vi "Collision detect speed test.vi"() -> ()   [LabVIEW 2024]
panel:
  in  "stop":bool
  out "Hz":dbl
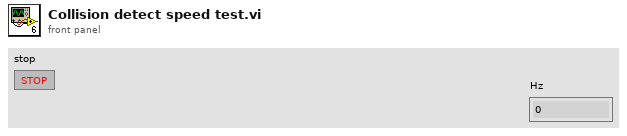
[diagram p1: front panel]
types:
  T1 = cluster{"X":dbl, "Y":dbl, "Object type":dbl, "Move info":dbl, "Vector scalar":dbl, "Vector theta":dbl}
  T2 = cluster{"X":dbl, "Y":dbl, "Object type":dbl, "Radius":dbl, "Width":dbl, "Height":dbl, "Theta":dbl, "HP":dbl, "R":dbl, "G":dbl, "B":dbl}[]
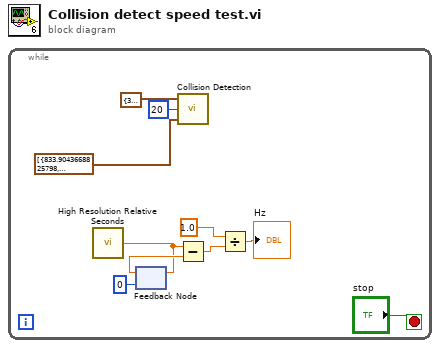
[diagram p0: block diagram]
diagram:
  n1 = while {
    stop <- "stop" stop-if-true
    n2 = call <vilib>:"High Resolution Relative Seconds.vi"() -> ("relative seconds"=w5:dbl)
    n3 = feedback #1(u32 0 ("millisecond timer value")) -> (w6:dbl)
    n4 = feedback-in #1(w5) -> ()
    n5 = call "Collision Detection.vi"("Map Entity Objects Positions"=T2 [{"X"=833.9043668825798, "Y"=359.94566828958796, "Object type"=0.0, "Radius"=30.0, "Width"=0.0, "Height"=0.0, "Theta"=5.711847827345959, "HP"=300.0, "R"=0.0, "G"=0.0, "B"=0.0}, {"X"=2580.0, "Y"=150.0, "Object type"=0.0, "Radius"=30.0, "Width"=0.0, "Height"=0.0, "Theta"=0.0, "HP"=300.0, "R"=0.0, "G"=0.0, "B"=0.0}, {"X"=1470.0, "Y"=390.0, "Object type"=0.0, "Radius"=30.0, "Width"=0.0, "Height"=0.0, "Theta"=0.0, "HP"=300.0, "R"=0.0, "G"=0.0, "B"=0.0}, {"X"=3690.0, "Y"=450.0, "Object type"=0.0, "Radius"=30.0, "Width"=0.0, "Height"=0.0, "Theta"=0.0, "HP"=300.0, "R"=0.0, "G"=0.0, "B"=0.0}, {"X"=2970.0, "Y"=690.0, "Object type"=0.0, "Radius"=30.0, "Width"=0.0, "Height"=0.0, "Theta"=0.0, "HP"=300.0, "R"=0.0, "G"=0.0, "B"=0.0}, {"X"=2130.0, "Y"=750.0, "Object type"=0.0, "Radius"=30.0, "Width"=0.0, "Height"=0.0, "Theta"=0.0, "HP"=300.0, "R"=0.0, "G"=0.0, "B"=0.0}, {"X"=150.0, "Y"=810.0, "Object type"=0.0, "Radius"=30.0, "Width"=0.0, "Height"=0.0, "Theta"=0.0, "HP"=300.0, "R"=0.0, "G"=0.0, "B"=0.0}, {"X"=1290.0, "Y"=1170.0, "Object type"=0.0, "Radius"=30.0, "Width"=0.0, "Height"=0.0, "Theta"=0.0, "HP"=300.0, "R"=0.0, "G"=0.0, "B"=0.0}, {"X"=390.0, "Y"=1290.0, "Object type"=0.0, "Radius"=30.0, "Width"=0.0, "Height"=0.0, "Theta"=0.0, "HP"=300.0, "R"=0.0, "G"=0.0, "B"=0.0}, {"X"=3210.0, "Y"=1290.0, "Object type"=0.0, "Radius"=30.0, "Width"=0.0, "Height"=0.0, "Theta"=0.0, "HP"=300.0, "R"=0.0, "G"=0.0, "B"=0.0}, {"X"=1950.0, "Y"=1710.0, "Object type"=0.0, "Radius"=30.0, "Width"=0.0, "Height"=0.0, "Theta"=0.0, "HP"=300.0, "R"=0.0, "G"=0.0, "B"=0.0}, {"X"=210.0, "Y"=1890.0, "Object type"=0.0, "Radius"=30.0, "Width"=0.0, "Height"=0.0, "Theta"=0.0, "HP"=300.0, "R"=0.0, "G"=0.0, "B"=0.0}, {"X"=2430.0, "Y"=2010.0, "Object type"=0.0, "Radius"=30.0, "Width"=0.0, "Height"=0.0, "Theta"=0.0, "HP"=300.0, "R"=0.0, "G"=0.0, "B"=0.0}, {"X"=3510.0, "Y"=2220.0, "Object type"=0.0, "Radius"=30.0, "Width"=0.0, "Height"=0.0, "Theta"=0.0, "HP"=300.0, "R"=0.0, "G"=0.0, "B"=0.0}, {"X"=1350.0, "Y"=2340.0, "Object type"=0.0, "Radius"=30.0, "Width"=0.0, "Height"=0.0, "Theta"=0.0, "HP"=300.0, "R"=0.0, "G"=0.0, "B"=0.0}, {"X"=330.0, "Y"=2730.0, "Object type"=0.0, "Radius"=30.0, "Width"=0.0, "Height"=0.0, "Theta"=0.0, "HP"=300.0, "R"=0.0, "G"=0.0, "B"=0.0}, {"X"=2790.0, "Y"=2790.0, "Object type"=0.0, "Radius"=30.0, "Width"=0.0, "Height"=0.0, "Theta"=0.0, "HP"=300.0, "R"=0.0, "G"=0.0, "B"=0.0}, {"X"=1950.0, "Y"=3150.0, "Object type"=0.0, "Radius"=30.0, "Width"=0.0, "Height"=0.0, "Theta"=0.0, "HP"=300.0, "R"=0.0, "G"=0.0, "B"=0.0}, {"X"=3330.0, "Y"=3390.0, "Object type"=0.0, "Radius"=30.0, "Width"=0.0, "Height"=0.0, "Theta"=0.0, "HP"=300.0, "R"=0.0, "G"=0.0, "B"=0.0}, {"X"=990.0, "Y"=3450.0, "Object type"=0.0, "Radius"=30.0, "Width"=0.0, "Height"=0.0, "Theta"=0.0, "HP"=300.0, "R"=0.0, "G"=0.0, "B"=0.0}, {"X"=630.0, "Y"=510.0, "Object type"=3.0, "Radius"=47.0, "Width"=0.0, "Height"=0.0, "Theta"=0.0, "HP"=-1000.0, "R"=0.0, "G"=85.0, "B"=0.0}, {"X"=1540.0, "Y"=1054.0, "Object type"=3.0, "Radius"=86.0, "Width"=0.0, "Height"=0.0, "Theta"=0.0, "HP"=-1000.0, "R"=0.0, "G"=85.0, "B"=0.0}, {"X"=1060.0, "Y"=200.0, "Object type"=3.0, "Radius"=72.0, "Width"=0.0, "Height"=0.0, "Theta"=0.0, "HP"=-1000.0, "R"=0.0, "G"=85.0, "B"=0.0}, {"X"=200.0, "Y"=460.0, "Object type"=3.0, "Radius"=62.0, "Width"=0.0, "Height"=0.0, "Theta"=0.0, "HP"=-1000.0, "R"=0.0, "G"=85.0, "B"=0.0}, {"X"=925.0, "Y"=990.0, "Object type"=3.0, "Radius"=68.0, "Width"=0.0, "Height"=0.0, "Theta"=0.0, "HP"=-1000.0, "R"=0.0, "G"=85.0, "B"=0.0}, {"X"=324.0, "Y"=846.0, "Object type"=3.0, "Radius"=73.0, "Width"=0.0, "Height"=0.0, "Theta"=0.0, "HP"=-1000.0, "R"=0.0, "G"=85.0, "B"=0.0}, {"X"=589.0, "Y"=1476.0, "Object type"=3.0, "Radius"=54.0, "Width"=0.0, "Height"=0.0, "Theta"=0.0, "HP"=-1000.0, "R"=0.0, "G"=85.0, "B"=0.0}, {"X"=1650.0, "Y"=1590.0, "Object type"=3.0, "Radius"=60.0, "Width"=0.0, "Height"=0.0, "Theta"=0.0, "HP"=-1000.0, "R"=0.0, "G"=85.0, "B"=0.0}, {"X"=2150.0, "Y"=1590.0, "Object type"=3.0, "Radius"=50.0, "Width"=0.0, "Height"=0.0, "Theta"=0.0, "HP"=-1000.0, "R"=0.0, "G"=85.0, "B"=0.0}, {"X"=990.0, "Y"=690.0, "Object type"=3.0, "Radius"=65.0, "Width"=0.0, "Height"=0.0, "Theta"=0.0, "HP"=-1000.0, "R"=0.0, "G"=85.0, "B"=0.0}, {"X"=1830.0, "Y"=390.0, "Object type"=3.0, "Radius"=73.0, "Width"=0.0, "Height"=0.0, "Theta"=0.0, "HP"=-1000.0, "R"=0.0, "G"=85.0, "B"=0.0}, {"X"=1770.0, "Y"=570.0, "Object type"=3.0, "Radius"=83.0, "Width"=0.0, "Height"=0.0, "Theta"=0.0, "HP"=-1000.0, "R"=0.0, "G"=85.0, "B"=0.0}, {"X"=1950.0, "Y"=510.0, "Object type"=3.0, "Radius"=80.0, "Width"=0.0, "Height"=0.0, "Theta"=0.0, "HP"=-1000.0, "R"=0.0, "G"=85.0, "B"=0.0}, {"X"=201.0, "Y"=140.0, "Object type"=3.0, "Radius"=35.0, "Width"=0.0, "Height"=0.0, "Theta"=0.0, "HP"=-1000.0, "R"=0.0, "G"=255.0, "B"=36.0}, {"X"=340.0, "Y"=160.0, "Object type"=3.0, "Radius"=40.0, "Width"=0.0, "Height"=0.0, "Theta"=0.0, "HP"=-1000.0, "R"=0.0, "G"=255.0, "B"=36.0}, {"X"=2398.0, "Y"=165.0, "Object type"=3.0, "Radius"=37.0, "Width"=0.0, "Height"=0.0, "Theta"=0.0, "HP"=-1000.0, "R"=0.0, "G"=255.0, "B"=36.0}, {"X"=627.0, "Y"=744.0, "Object type"=3.0, "Radius"=21.0, "Width"=0.0, "Height"=0.0, "Theta"=0.0, "HP"=-1000.0, "R"=0.0, "G"=255.0, "B"=36.0}, {"X"=3302.0, "Y"=167.0, "Object type"=3.0, "Radius"=26.0, "Width"=0.0, "Height"=0.0, "Theta"=0.0, "HP"=-1000.0, "R"=0.0, "G"=255.0, "B"=36.0}, {"X"=3587.0, "Y"=199.0, "Object type"=3.0, "Radius"=41.0, "Width"=0.0, "Height"=0.0, "Theta"=0.0, "HP"=-1000.0, "R"=0.0, "G"=255.0, "B"=36.0}, {"X"=3204.0, "Y"=641.0, "Object type"=3.0, "Radius"=33.0, "Width"=0.0, "Height"=0.0, "Theta"=0.0, "HP"=-1000.0, "R"=0.0, "G"=255.0, "B"=36.0}, {"X"=2563.0, "Y"=681.0, "Object type"=3.0, "Radius"=28.0, "Width"=0.0, "Height"=0.0, "Theta"=0.0, "HP"=-1000.0, "R"=0.0, "G"=255.0, "B"=36.0}, {"X"=2913.0, "Y"=867.0, "Object type"=3.0, "Radius"=52.0, "Width"=0.0, "Height"=0.0, "Theta"=0.0, "HP"=-1000.0, "R"=0.0, "G"=255.0, "B"=36.0}, {"X"=3411.0, "Y"=1021.0, "Object type"=3.0, "Radius"=85.0, "Width"=0.0, "Height"=0.0, "Theta"=0.0, "HP"=-1000.0, "R"=0.0, "G"=255.0, "B"=36.0}, {"X"=2453.0, "Y"=941.0, "Object type"=3.0, "Radius"=35.0, "Width"=0.0, "Height"=0.0, "Theta"=0.0, "HP"=-1000.0, "R"=0.0, "G"=255.0, "B"=36.0}, {"X"=2193.0, "Y"=1012.0, "Object type"=3.0, "Radius"=24.0, "Width"=0.0, "Height"=0.0, "Theta"=0.0, "HP"=-1000.0, "R"=179.0, "G"=255.0, "B"=42.0}, {"X"=2134.0, "Y"=1254.0, "Object type"=3.0, "Radius"=34.0, "Width"=0.0, "Height"=0.0, "Theta"=0.0, "HP"=-1000.0, "R"=179.0, "G"=255.0, "B"=42.0}, {"X"=881.0, "Y"=1245.0, "Object type"=3.0, "Radius"=28.0, "Width"=0.0, "Height"=0.0, "Theta"=0.0, "HP"=-1000.0, "R"=179.0, "G"=255.0, "B"=42.0}, {"X"=1000.0, "Y"=1369.0, "Object type"=3.0, "Radius"=32.0, "Width"=0.0, "Height"=0.0, "Theta"=0.0, "HP"=-1000.0, "R"=0.0, "G"=255.0, "B"=36.0}, {"X"=1151.0, "Y"=1489.0, "Object type"=3.0, "Radius"=36.0, "Width"=0.0, "Height"=0.0, "Theta"=0.0, "HP"=-1000.0, "R"=179.0, "G"=255.0, "B"=42.0}, {"X"=399.0, "Y"=1632.0, "Object type"=3.0, "Radius"=28.0, "Width"=0.0, "Height"=0.0, "Theta"=0.0, "HP"=-1000.0, "R"=179.0, "G"=255.0, "B"=42.0}, {"X"=671.0, "Y"=1711.0, "Object type"=3.0, "Radius"=34.0, "Width"=0.0, "Height"=0.0, "Theta"=0.0, "HP"=-1000.0, "R"=179.0, "G"=255.0, "B"=42.0}, {"X"=1025.0, "Y"=1678.0, "Object type"=3.0, "Radius"=36.0, "Width"=0.0, "Height"=0.0, "Theta"=0.0, "HP"=-1000.0, "R"=0.0, "G"=255.0, "B"=36.0}, {"X"=145.0, "Y"=2031.0, "Object type"=3.0, "Radius"=41.0, "Width"=0.0, "Height"=0.0, "Theta"=0.0, "HP"=-1000.0, "R"=0.0, "G"=255.0, "B"=36.0}, {"X"=476.0, "Y"=1931.0, "Object type"=3.0, "Radius"=71.0, "Width"=0.0, "Height"=0.0, "Theta"=0.0, "HP"=-1000.0, "R"=0.0, "G"=255.0, "B"=36.0}, {"X"=756.0, "Y"=1999.0, "Object type"=3.0, "Radius"=29.0, "Width"=0.0, "Height"=0.0, "Theta"=0.0, "HP"=-1000.0, "R"=179.0, "G"=255.0, "B"=42.0}, {"X"=1113.0, "Y"=67.0, "Object type"=3.0, "Radius"=88.0, "Width"=0.0, "Height"=0.0, "Theta"=0.0, "HP"=-1000.0, "R"=0.0, "G"=255.0, "B"=36.0}, {"X"=504.0, "Y"=2241.0, "Object type"=3.0, "Radius"=37.0, "Width"=0.0, "Height"=0.0, "Theta"=0.0, "HP"=-1000.0, "R"=0.0, "G"=255.0, "B"=36.0}, {"X"=936.0, "Y"=2441.0, "Object type"=3.0, "Radius"=25.0, "Width"=0.0, "Height"=0.0, "Theta"=0.0, "HP"=-1000.0, "R"=179.0, "G"=255.0, "B"=42.0}, {"X"=587.0, "Y"=2753.0, "Object type"=3.0, "Radius"=27.0, "Width"=0.0, "Height"=0.0, "Theta"=0.0, "HP"=-1000.0, "R"=179.0, "G"=255.0, "B"=42.0}, {"X"=952.0, "Y"=2801.0, "Object type"=3.0, "Radius"=91.0, "Width"=0.0, "Height"=0.0, "Theta"=0.0, "HP"=-1000.0, "R"=0.0, "G"=255.0, "B"=36.0}, {"X"=134.0, "Y"=3078.0, "Object type"=3.0, "Radius"=67.0, "Width"=0.0, "Height"=0.0, "Theta"=0.0, "HP"=-1000.0, "R"=0.0, "G"=255.0, "B"=36.0}, {"X"=381.0, "Y"=3381.0, "Object type"=3.0, "Radius"=94.0, "Width"=0.0, "Height"=0.0, "Theta"=0.0, "HP"=-1000.0, "R"=179.0, "G"=255.0, "B"=42.0}, {"X"=659.0, "Y"=3549.0, "Object type"=3.0, "Radius"=83.0, "Width"=0.0, "Height"=0.0, "Theta"=0.0, "HP"=-1000.0, "R"=179.0, "G"=255.0, "B"=42.0}, {"X"=921.0, "Y"=3651.0, "Object type"=3.0, "Radius"=33.0, "Width"=0.0, "Height"=0.0, "Theta"=0.0, "HP"=-1000.0, "R"=0.0, "G"=255.0, "B"=36.0}, {"X"=1247.0, "Y"=3539.0, "Object type"=3.0, "Radius"=51.0, "Width"=0.0, "Height"=0.0, "Theta"=0.0, "HP"=-1000.0, "R"=179.0, "G"=255.0, "B"=42.0}, {"X"=1292.0, "Y"=3217.0, "Object type"=3.0, "Radius"=41.0, "Width"=0.0, "Height"=0.0, "Theta"=0.0, "HP"=-1000.0, "R"=0.0, "G"=255.0, "B"=36.0}, {"X"=1435.0, "Y"=2876.0, "Object type"=3.0, "Radius"=79.0, "Width"=0.0, "Height"=0.0, "Theta"=0.0, "HP"=-1000.0, "R"=179.0, "G"=255.0, "B"=42.0}, {"X"=1620.0, "Y"=2173.0, "Object type"=3.0, "Radius"=71.0, "Width"=0.0, "Height"=0.0, "Theta"=0.0, "HP"=-1000.0, "R"=0.0, "G"=255.0, "B"=36.0}, {"X"=1550.0, "Y"=1901.0, "Object type"=3.0, "Radius"=37.0, "Width"=0.0, "Height"=0.0, "Theta"=0.0, "HP"=-1000.0, "R"=0.0, "G"=255.0, "B"=36.0}, {"X"=2786.0, "Y"=1543.0, "Object type"=3.0, "Radius"=26.0, "Width"=0.0, "Height"=0.0, "Theta"=0.0, "HP"=-1000.0, "R"=179.0, "G"=255.0, "B"=42.0}, {"X"=3371.0, "Y"=1701.0, "Object type"=3.0, "Radius"=29.0, "Width"=0.0, "Height"=0.0, "Theta"=0.0, "HP"=-1000.0, "R"=0.0, "G"=255.0, "B"=36.0}, {"X"=3579.0, "Y"=1534.0, "Object type"=3.0, "Radius"=34.0, "Width"=0.0, "Height"=0.0, "Theta"=0.0, "HP"=-1000.0, "R"=179.0, "G"=255.0, "B"=42.0}, {"X"=2482.93, "Y"=321.21, "Object type"=4.0, "Radius"=0.0, "Width"=84.853, "Height"=20.0, "Theta"=2.356, "HP"=-1000.0, "R"=179.0, "G"=255.0, "B"=42.0}, {"X"=2437.07, "Y"=321.21, "Object type"=4.0, "Radius"=0.0, "Width"=84.853, "Height"=20.0, "Theta"=0.785, "HP"=-1000.0, "R"=179.0, "G"=255.0, "B"=42.0}, {"X"=2460.0, "Y"=390.0, "Object type"=4.0, "Radius"=0.0, "Width"=111.72, "Height"=20.0, "Theta"=2.356, "HP"=-1000.0, "R"=179.0, "G"=255.0, "B"=42.0}, {"X"=2482.93, "Y"=458.79, "Object type"=4.0, "Radius"=0.0, "Width"=84.853, "Height"=20.0, "Theta"=0.785, "HP"=-1000.0, "R"=179.0, "G"=255.0, "B"=42.0}, {"X"=2437.07, "Y"=458.79, "Object type"=4.0, "Radius"=0.0, "Width"=84.853, "Height"=20.0, "Theta"=2.356, "HP"=-1000.0, "R"=179.0, "G"=255.0, "B"=42.0}, {"X"=2640.0, "Y"=420.0, "Object type"=4.0, "Radius"=0.0, "Width"=100.0, "Height"=21.0, "Theta"=1.92, "HP"=-1000.0, "R"=179.0, "G"=255.0, "B"=42.0}, {"X"=2700.0, "Y"=420.0, "Object type"=4.0, "Radius"=0.0, "Width"=100.0, "Height"=21.0, "Theta"=1.22, "HP"=-1000.0, "R"=179.0, "G"=255.0, "B"=42.0}, {"X"=2891.0, "Y"=390.0, "Object type"=4.0, "Radius"=0.0, "Width"=120.0, "Height"=18.0, "Theta"=1.57, "HP"=-1000.0, "R"=179.0, "G"=255.0, "B"=42.0}, {"X"=2950.0, "Y"=390.0, "Object type"=4.0, "Radius"=0.0, "Width"=120.0, "Height"=18.0, "Theta"=2.01, "HP"=-1000.0, "R"=179.0, "G"=255.0, "B"=42.0}, {"X"=3060.0, "Y"=390.0, "Object type"=4.0, "Radius"=0.0, "Width"=180.28, "Height"=25.0, "Theta"=1.91, "HP"=-1000.0, "R"=179.0, "G"=255.0, "B"=42.0}, {"X"=3120.0, "Y"=390.0, "Object type"=4.0, "Radius"=0.0, "Width"=180.28, "Height"=25.0, "Theta"=1.23, "HP"=-1000.0, "R"=179.0, "G"=255.0, "B"=42.0}, {"X"=3420.0, "Y"=390.0, "Object type"=4.0, "Radius"=0.0, "Width"=180.28, "Height"=25.0, "Theta"=1.91, "HP"=-1000.0, "R"=179.0, "G"=255.0, "B"=42.0}, {"X"=3480.0, "Y"=390.0, "Object type"=4.0, "Radius"=0.0, "Width"=180.28, "Height"=25.0, "Theta"=1.23, "HP"=-1000.0, "R"=179.0, "G"=255.0, "B"=42.0}, {"X"=435.0, "Y"=260.0, "Object type"=1.0, "Radius"=25.0, "Width"=0.0, "Height"=0.0, "Theta"=0.0, "HP"=-1000.0, "R"=100.0, "G"=60.0, "B"=11.0}, {"X"=1060.0, "Y"=200.0, "Object type"=1.0, "Radius"=23.0, "Width"=0.0, "Height"=0.0, "Theta"=0.0, "HP"=-1000.0, "R"=100.0, "G"=60.0, "B"=11.0}, {"X"=1190.0, "Y"=450.0, "Object type"=1.0, "Radius"=40.0, "Width"=0.0, "Height"=0.0, "Theta"=0.0, "HP"=-1000.0, "R"=100.0, "G"=60.0, "B"=11.0}, {"X"=1300.0, "Y"=670.0, "Object type"=1.0, "Radius"=45.0, "Width"=0.0, "Height"=0.0, "Theta"=0.0, "HP"=-1000.0, "R"=100.0, "G"=60.0, "B"=11.0}, {"X"=200.0, "Y"=460.0, "Object type"=1.0, "Radius"=25.0, "Width"=0.0, "Height"=0.0, "Theta"=0.0, "HP"=-1000.0, "R"=100.0, "G"=60.0, "B"=11.0}, {"X"=630.0, "Y"=470.0, "Object type"=1.0, "Radius"=27.0, "Width"=0.0, "Height"=0.0, "Theta"=0.0, "HP"=-1000.0, "R"=100.0, "G"=60.0, "B"=11.0}, {"X"=575.0, "Y"=543.0, "Object type"=1.0, "Radius"=29.0, "Width"=0.0, "Height"=0.0, "Theta"=0.0, "HP"=-1000.0, "R"=100.0, "G"=60.0, "B"=11.0}, {"X"=660.0, "Y"=554.0, "Object type"=1.0, "Radius"=16.0, "Width"=0.0, "Height"=0.0, "Theta"=0.0, "HP"=-1000.0, "R"=100.0, "G"=60.0, "B"=11.0}, {"X"=329.0, "Y"=846.0, "Object type"=1.0, "Radius"=34.0, "Width"=0.0, "Height"=0.0, "Theta"=0.0, "HP"=-1000.0, "R"=100.0, "G"=60.0, "B"=11.0}, {"X"=621.0, "Y"=883.0, "Object type"=1.0, "Radius"=21.0, "Width"=0.0, "Height"=0.0, "Theta"=0.0, "HP"=-1000.0, "R"=100.0, "G"=60.0, "B"=11.0}, {"X"=925.0, "Y"=990.0, "Object type"=1.0, "Radius"=34.0, "Width"=0.0, "Height"=0.0, "Theta"=0.0, "HP"=-1000.0, "R"=100.0, "G"=60.0, "B"=11.0}, {"X"=1540.0, "Y"=1054.0, "Object type"=1.0, "Radius"=38.0, "Width"=0.0, "Height"=0.0, "Theta"=0.0, "HP"=-1000.0, "R"=100.0, "G"=60.0, "B"=11.0}, {"X"=2940.0, "Y"=145.0, "Object type"=1.0, "Radius"=48.0, "Width"=0.0, "Height"=0.0, "Theta"=0.0, "HP"=-1000.0, "R"=100.0, "G"=60.0, "B"=11.0}, {"X"=167.0, "Y"=1403.0, "Object type"=1.0, "Radius"=29.0, "Width"=0.0, "Height"=0.0, "Theta"=0.0, "HP"=-1000.0, "R"=100.0, "G"=60.0, "B"=11.0}, {"X"=589.0, "Y"=1476.0, "Object type"=1.0, "Radius"=29.0, "Width"=0.0, "Height"=0.0, "Theta"=0.0, "HP"=-1000.0, "R"=100.0, "G"=60.0, "B"=11.0}, {"X"=1650.0, "Y"=1590.0, "Object type"=1.0, "Radius"=27.0, "Width"=0.0, "Height"=0.0, "Theta"=0.0, "HP"=-1000.0, "R"=100.0, "G"=60.0, "B"=11.0}, {"X"=2150.0, "Y"=1950.0, "Object type"=1.0, "Radius"=18.0, "Width"=0.0, "Height"=0.0, "Theta"=0.0, "HP"=-1000.0, "R"=100.0, "G"=60.0, "B"=11.0}, {"X"=1173.0, "Y"=1783.0, "Object type"=1.0, "Radius"=24.0, "Width"=0.0, "Height"=0.0, "Theta"=0.0, "HP"=-1000.0, "R"=100.0, "G"=60.0, "B"=11.0}, {"X"=2261.0, "Y"=1563.0, "Object type"=1.0, "Radius"=31.0, "Width"=0.0, "Height"=0.0, "Theta"=0.0, "HP"=-1000.0, "R"=100.0, "G"=60.0, "B"=11.0}, {"X"=990.0, "Y"=690.0, "Object type"=1.0, "Radius"=32.0, "Width"=0.0, "Height"=0.0, "Theta"=0.0, "HP"=-1000.0, "R"=100.0, "G"=60.0, "B"=11.0}, {"X"=1830.0, "Y"=390.0, "Object type"=1.0, "Radius"=28.0, "Width"=0.0, "Height"=0.0, "Theta"=0.0, "HP"=-1000.0, "R"=100.0, "G"=60.0, "B"=11.0}, {"X"=1770.0, "Y"=570.0, "Object type"=1.0, "Radius"=33.0, "Width"=0.0, "Height"=0.0, "Theta"=0.0, "HP"=-1000.0, "R"=100.0, "G"=60.0, "B"=11.0}, {"X"=1950.0, "Y"=510.0, "Object type"=1.0, "Radius"=36.0, "Width"=0.0, "Height"=0.0, "Theta"=0.0, "HP"=-1000.0, "R"=100.0, "G"=60.0, "B"=11.0}, {"X"=1973.0, "Y"=1121.0, "Object type"=1.0, "Radius"=40.0, "Width"=0.0, "Height"=0.0, "Theta"=0.0, "HP"=-1000.0, "R"=100.0, "G"=60.0, "B"=11.0}, {"X"=2910.0, "Y"=330.0, "Object type"=1.0, "Radius"=28.0, "Width"=0.0, "Height"=0.0, "Theta"=0.0, "HP"=-1000.0, "R"=100.0, "G"=100.0, "B"=100.0}, {"X"=2670.0, "Y"=450.0, "Object type"=1.0, "Radius"=27.0, "Width"=0.0, "Height"=0.0, "Theta"=0.0, "HP"=-1000.0, "R"=100.0, "G"=100.0, "B"=100.0}, {"X"=2173.0, "Y"=378.0, "Object type"=1.0, "Radius"=26.0, "Width"=0.0, "Height"=0.0, "Theta"=0.0, "HP"=-1000.0, "R"=151.0, "G"=151.0, "B"=151.0}, {"X"=3451.0, "Y"=681.0, "Object type"=1.0, "Radius"=32.0, "Width"=0.0, "Height"=0.0, "Theta"=0.0, "HP"=-1000.0, "R"=151.0, "G"=151.0, "B"=151.0}, {"X"=2583.0, "Y"=2927.0, "Object type"=1.0, "Radius"=70.0, "Width"=0.0, "Height"=0.0, "Theta"=0.0, "HP"=-1000.0, "R"=100.0, "G"=100.0, "B"=100.0}, {"X"=2188.0, "Y"=2674.0, "Object type"=1.0, "Radius"=26.0, "Width"=0.0, "Height"=0.0, "Theta"=0.0, "HP"=-1000.0, "R"=151.0, "G"=151.0, "B"=151.0}, {"X"=373.0, "Y"=2539.0, "Object type"=1.0, "Radius"=19.0, "Width"=0.0, "Height"=0.0, "Theta"=0.0, "HP"=-1000.0, "R"=151.0, "G"=151.0, "B"=151.0}, {"X"=256.0, "Y"=2873.0, "Object type"=1.0, "Radius"=14.0, "Width"=0.0, "Height"=0.0, "Theta"=0.0, "HP"=-1000.0, "R"=100.0, "G"=100.0, "B"=100.0}, {"X"=2494.0, "Y"=1248.0, "Object type"=1.0, "Radius"=27.0, "Width"=0.0, "Height"=0.0, "Theta"=0.0, "HP"=-1000.0, "R"=151.0, "G"=151.0, "B"=151.0}, {"X"=814.0, "Y"=2256.0, "Object type"=1.0, "Radius"=45.0, "Width"=0.0, "Height"=0.0, "Theta"=0.0, "HP"=-1000.0, "R"=151.0, "G"=151.0, "B"=151.0}, {"X"=1111.0, "Y"=3345.0, "Object type"=1.0, "Radius"=34.0, "Width"=0.0, "Height"=0.0, "Theta"=0.0, "HP"=-1000.0, "R"=100.0, "G"=100.0, "B"=100.0}, {"X"=3397.0, "Y"=3513.0, "Object type"=2.0, "Radius"=0.0, "Width"=140.0, "Height"=24.0, "Theta"=0.0, "HP"=-1000.0, "R"=100.0, "G"=100.0, "B"=100.0}, {"X"=3510.0, "Y"=3456.0, "Object type"=2.0, "Radius"=0.0, "Width"=120.0, "Height"=37.0, "Theta"=0.96, "HP"=-1000.0, "R"=100.0, "G"=100.0, "B"=100.0}, {"X"=3176.0, "Y"=3238.0, "Object type"=2.0, "Radius"=0.0, "Width"=137.0, "Height"=29.0, "Theta"=0.0, "HP"=-1000.0, "R"=151.0, "G"=151.0, "B"=151.0}, {"X"=3382.0, "Y"=3098.0, "Object type"=2.0, "Radius"=0.0, "Width"=163.0, "Height"=33.0, "Theta"=2.18, "HP"=-1000.0, "R"=100.0, "G"=100.0, "B"=100.0}, {"X"=3340.0, "Y"=2120.0, "Object type"=2.0, "Radius"=0.0, "Width"=140.0, "Height"=40.0, "Theta"=1.57, "HP"=-1000.0, "R"=100.0, "G"=100.0, "B"=100.0}, {"X"=3340.0, "Y"=2240.0, "Object type"=2.0, "Radius"=0.0, "Width"=100.0, "Height"=40.0, "Theta"=1.57, "HP"=-1000.0, "R"=100.0, "G"=100.0, "B"=100.0}, {"X"=2140.0, "Y"=1980.0, "Object type"=2.0, "Radius"=0.0, "Width"=160.0, "Height"=20.0, "Theta"=0.0, "HP"=-1000.0, "R"=100.0, "G"=100.0, "B"=100.0}, {"X"=2080.0, "Y"=1960.0, "Object type"=2.0, "Radius"=0.0, "Width"=160.0, "Height"=20.0, "Theta"=1.57, "HP"=-1000.0, "R"=100.0, "G"=100.0, "B"=100.0}, {"X"=2160.0, "Y"=2020.0, "Object type"=2.0, "Radius"=0.0, "Width"=160.0, "Height"=20.0, "Theta"=0.0, "HP"=-1000.0, "R"=100.0, "G"=100.0, "B"=100.0}, {"X"=2220.0, "Y"=1940.0, "Object type"=2.0, "Radius"=0.0, "Width"=160.0, "Height"=20.0, "Theta"=1.57, "HP"=-1000.0, "R"=100.0, "G"=100.0, "B"=100.0}, {"X"=1592.66, "Y"=1549.85, "Object type"=2.0, "Radius"=0.0, "Width"=160.0, "Height"=20.0, "Theta"=0.96, "HP"=-1000.0, "R"=100.0, "G"=100.0, "B"=100.0}, {"X"=1609.85, "Y"=1647.34, "Object type"=2.0, "Radius"=0.0, "Width"=160.0, "Height"=20.0, "Theta"=2.53, "HP"=-1000.0, "R"=100.0, "G"=100.0, "B"=100.0}, {"X"=1707.34, "Y"=1630.15, "Object type"=2.0, "Radius"=0.0, "Width"=160.0, "Height"=20.0, "Theta"=0.96, "HP"=-1000.0, "R"=100.0, "G"=100.0, "B"=100.0}, {"X"=1690.15, "Y"=1532.66, "Object type"=2.0, "Radius"=0.0, "Width"=160.0, "Height"=20.0, "Theta"=2.53, "HP"=-1000.0, "R"=100.0, "G"=100.0, "B"=100.0}, {"X"=2910.0, "Y"=3150.0, "Object type"=2.0, "Radius"=0.0, "Width"=180.0, "Height"=35.0, "Theta"=1.57, "HP"=-1000.0, "R"=151.0, "G"=151.0, "B"=151.0}, {"X"=2910.0, "Y"=3330.0, "Object type"=2.0, "Radius"=0.0, "Width"=180.0, "Height"=35.0, "Theta"=1.57, "HP"=-1000.0, "R"=151.0, "G"=151.0, "B"=151.0}, {"X"=2600.0, "Y"=3500.0, "Object type"=2.0, "Radius"=0.0, "Width"=170.0, "Height"=25.0, "Theta"=1.8, "HP"=-1000.0, "R"=100.0, "G"=100.0, "B"=100.0}, {"X"=2300.0, "Y"=3535.0, "Object type"=2.0, "Radius"=0.0, "Width"=190.0, "Height"=30.0, "Theta"=0.4, "HP"=-1000.0, "R"=151.0, "G"=151.0, "B"=151.0}, {"X"=2000.0, "Y"=3640.0, "Object type"=2.0, "Radius"=0.0, "Width"=185.0, "Height"=27.0, "Theta"=1.34, "HP"=-1000.0, "R"=100.0, "G"=100.0, "B"=100.0}, {"X"=1730.0, "Y"=3170.0, "Object type"=2.0, "Radius"=0.0, "Width"=195.0, "Height"=33.0, "Theta"=1.77, "HP"=-1000.0, "R"=100.0, "G"=100.0, "B"=100.0}, {"X"=3140.0, "Y"=2785.0, "Object type"=2.0, "Radius"=0.0, "Width"=158.0, "Height"=18.0, "Theta"=1.64, "HP"=-1000.0, "R"=151.0, "G"=151.0, "B"=151.0}, {"X"=2650.0, "Y"=2485.0, "Object type"=2.0, "Radius"=0.0, "Width"=200.0, "Height"=40.0, "Theta"=6.0, "HP"=-1000.0, "R"=100.0, "G"=100.0, "B"=100.0}, {"X"=3014.0, "Y"=2178.0, "Object type"=2.0, "Radius"=0.0, "Width"=175.0, "Height"=22.0, "Theta"=1.14, "HP"=-1000.0, "R"=100.0, "G"=100.0, "B"=100.0}, {"X"=1966.0, "Y"=2498.0, "Object type"=2.0, "Radius"=0.0, "Width"=190.0, "Height"=25.0, "Theta"=1.6, "HP"=-1000.0, "R"=151.0, "G"=151.0, "B"=151.0}, {"X"=867.0, "Y"=3098.0, "Object type"=2.0, "Radius"=0.0, "Width"=187.0, "Height"=24.0, "Theta"=5.91, "HP"=-1000.0, "R"=100.0, "G"=100.0, "B"=100.0}, {"X"=3054.0, "Y"=1154.0, "Object type"=2.0, "Radius"=0.0, "Width"=160.0, "Height"=38.0, "Theta"=5.8, "HP"=-1000.0, "R"=100.0, "G"=100.0, "B"=100.0}, {"X"=3324.0, "Y"=1503.0, "Object type"=2.0, "Radius"=0.0, "Width"=150.0, "Height"=20.0, "Theta"=0.61, "HP"=-1000.0, "R"=151.0, "G"=151.0, "B"=151.0}, {"X"=2301.0, "Y"=3504.0, "Object type"=2.0, "Radius"=0.0, "Width"=145.0, "Height"=24.0, "Theta"=0.85, "HP"=-1000.0, "R"=151.0, "G"=151.0, "B"=151.0}, {"X"=100.0, "Y"=10.0, "Object type"=2.0, "Radius"=0.0, "Width"=200.0, "Height"=20.0, "Theta"=0.0, "HP"=-1000.0, "R"=100.0, "G"=100.0, "B"=100.0}, {"X"=300.0, "Y"=10.0, "Object type"=2.0, "Radius"=0.0, "Width"=200.0, "Height"=20.0, "Theta"=0.0, "HP"=-1000.0, "R"=100.0, "G"=100.0, "B"=100.0}, {"X"=500.0, "Y"=10.0, "Object type"=2.0, "Radius"=0.0, "Width"=200.0, "Height"=20.0, "Theta"=0.0, "HP"=-1000.0, "R"=100.0, "G"=100.0, "B"=100.0}, {"X"=700.0, "Y"=10.0, "Object type"=2.0, "Radius"=0.0, "Width"=200.0, "Height"=20.0, "Theta"=0.0, "HP"=-1000.0, "R"=100.0, "G"=100.0, "B"=100.0}, {"X"=900.0, "Y"=10.0, "Object type"=2.0, "Radius"=0.0, "Width"=200.0, "Height"=20.0, "Theta"=0.0, "HP"=-1000.0, "R"=100.0, "G"=100.0, "B"=100.0}, {"X"=1100.0, "Y"=10.0, "Object type"=2.0, "Radius"=0.0, "Width"=200.0, "Height"=20.0, "Theta"=0.0, "HP"=-1000.0, "R"=100.0, "G"=100.0, "B"=100.0}, {"X"=1300.0, "Y"=10.0, "Object type"=2.0, "Radius"=0.0, "Width"=200.0, "Height"=20.0, "Theta"=0.0, "HP"=-1000.0, "R"=100.0, "G"=100.0, "B"=100.0}, {"X"=1500.0, "Y"=10.0, "Object type"=2.0, "Radius"=0.0, "Width"=200.0, "Height"=20.0, "Theta"=0.0, "HP"=-1000.0, "R"=100.0, "G"=100.0, "B"=100.0}, {"X"=1700.0, "Y"=10.0, "Object type"=2.0, "Radius"=0.0, "Width"=200.0, "Height"=20.0, "Theta"=0.0, "HP"=-1000.0, "R"=100.0, "G"=100.0, "B"=100.0}, {"X"=1900.0, "Y"=10.0, "Object type"=2.0, "Radius"=0.0, "Width"=200.0, "Height"=20.0, "Theta"=0.0, "HP"=-1000.0, "R"=100.0, "G"=100.0, "B"=100.0}, {"X"=2100.0, "Y"=10.0, "Object type"=2.0, "Radius"=0.0, "Width"=200.0, "Height"=20.0, "Theta"=0.0, "HP"=-1000.0, "R"=100.0, "G"=100.0, "B"=100.0}, {"X"=2300.0, "Y"=10.0, "Object type"=2.0, "Radius"=0.0, "Width"=200.0, "Height"=20.0, "Theta"=0.0, "HP"=-1000.0, "R"=100.0, "G"=100.0, "B"=100.0}, {"X"=2500.0, "Y"=10.0, "Object type"=2.0, "Radius"=0.0, "Width"=200.0, "Height"=20.0, "Theta"=0.0, "HP"=-1000.0, "R"=100.0, "G"=100.0, "B"=100.0}, {"X"=2700.0, "Y"=10.0, "Object type"=2.0, "Radius"=0.0, "Width"=200.0, "Height"=20.0, "Theta"=0.0, "HP"=-1000.0, "R"=100.0, "G"=100.0, "B"=100.0}, {"X"=2900.0, "Y"=10.0, "Object type"=2.0, "Radius"=0.0, "Width"=200.0, "Height"=20.0, "Theta"=0.0, "HP"=-1000.0, "R"=100.0, "G"=100.0, "B"=100.0}, {"X"=3100.0, "Y"=10.0, "Object type"=2.0, "Radius"=0.0, "Width"=200.0, "Height"=20.0, "Theta"=0.0, "HP"=-1000.0, "R"=100.0, "G"=100.0, "B"=100.0}, {"X"=3300.0, "Y"=10.0, "Object type"=2.0, "Radius"=0.0, "Width"=200.0, "Height"=20.0, "Theta"=0.0, "HP"=-1000.0, "R"=100.0, "G"=100.0, "B"=100.0}, {"X"=3500.0, "Y"=10.0, "Object type"=2.0, "Radius"=0.0, "Width"=200.0, "Height"=20.0, "Theta"=0.0, "HP"=-1000.0, "R"=100.0, "G"=100.0, "B"=100.0}, {"X"=3700.0, "Y"=10.0, "Object type"=2.0, "Radius"=0.0, "Width"=200.0, "Height"=20.0, "Theta"=0.0, "HP"=-1000.0, "R"=100.0, "G"=100.0, "B"=100.0}, {"X"=3900.0, "Y"=10.0, "Object type"=2.0, "Radius"=0.0, "Width"=200.0, "Height"=20.0, "Theta"=0.0, "HP"=-1000.0, "R"=100.0, "G"=100.0, "B"=100.0}, {"X"=100.0, "Y"=3830.0, "Object type"=2.0, "Radius"=0.0, "Width"=200.0, "Height"=20.0, "Theta"=0.0, "HP"=-1000.0, "R"=100.0, "G"=100.0, "B"=100.0}, {"X"=300.0, "Y"=3830.0, "Object type"=2.0, "Radius"=0.0, "Width"=200.0, "Height"=20.0, "Theta"=0.0, "HP"=-1000.0, "R"=100.0, "G"=100.0, "B"=100.0}, {"X"=500.0, "Y"=3830.0, "Object type"=2.0, "Radius"=0.0, "Width"=200.0, "Height"=20.0, "Theta"=0.0, "HP"=-1000.0, "R"=100.0, "G"=100.0, "B"=100.0}, {"X"=700.0, "Y"=3830.0, "Object type"=2.0, "Radius"=0.0, "Width"=200.0, "Height"=20.0, "Theta"=0.0, "HP"=-1000.0, "R"=100.0, "G"=100.0, "B"=100.0}, {"X"=900.0, "Y"=3830.0, "Object type"=2.0, "Radius"=0.0, "Width"=200.0, "Height"=20.0, "Theta"=0.0, "HP"=-1000.0, "R"=100.0, "G"=100.0, "B"=100.0}, {"X"=1100.0, "Y"=3830.0, "Object type"=2.0, "Radius"=0.0, "Width"=200.0, "Height"=20.0, "Theta"=0.0, "HP"=-1000.0, "R"=100.0, "G"=100.0, "B"=100.0}, {"X"=1300.0, "Y"=3830.0, "Object type"=2.0, "Radius"=0.0, "Width"=200.0, "Height"=20.0, "Theta"=0.0, "HP"=-1000.0, "R"=100.0, "G"=100.0, "B"=100.0}, {"X"=1500.0, "Y"=3830.0, "Object type"=2.0, "Radius"=0.0, "Width"=200.0, "Height"=20.0, "Theta"=0.0, "HP"=-1000.0, "R"=100.0, "G"=100.0, "B"=100.0}, {"X"=1700.0, "Y"=3830.0, "Object type"=2.0, "Radius"=0.0, "Width"=200.0, "Height"=20.0, "Theta"=0.0, "HP"=-1000.0, "R"=100.0, "G"=100.0, "B"=100.0}, {"X"=1900.0, "Y"=3830.0, "Object type"=2.0, "Radius"=0.0, "Width"=200.0, "Height"=20.0, "Theta"=0.0, "HP"=-1000.0, "R"=100.0, "G"=100.0, "B"=100.0}, {"X"=2100.0, "Y"=3830.0, "Object type"=2.0, "Radius"=0.0, "Width"=200.0, "Height"=20.0, "Theta"=0.0, "HP"=-1000.0, "R"=100.0, "G"=100.0, "B"=100.0}, {"X"=2300.0, "Y"=3830.0, "Object type"=2.0, "Radius"=0.0, "Width"=200.0, "Height"=20.0, "Theta"=0.0, "HP"=-1000.0, "R"=100.0, "G"=100.0, "B"=100.0}, {"X"=2500.0, "Y"=3830.0, "Object type"=2.0, "Radius"=0.0, "Width"=200.0, "Height"=20.0, "Theta"=0.0, "HP"=-1000.0, "R"=100.0, "G"=100.0, "B"=100.0}, {"X"=2700.0, "Y"=3830.0, "Object type"=2.0, "Radius"=0.0, "Width"=200.0, "Height"=20.0, "Theta"=0.0, "HP"=-1000.0, "R"=100.0, "G"=100.0, "B"=100.0}, {"X"=2900.0, "Y"=3830.0, "Object type"=2.0, "Radius"=0.0, "Width"=200.0, "Height"=20.0, "Theta"=0.0, "HP"=-1000.0, "R"=100.0, "G"=100.0, "B"=100.0}, {"X"=3100.0, "Y"=3830.0, "Object type"=2.0, "Radius"=0.0, "Width"=200.0, "Height"=20.0, "Theta"=0.0, "HP"=-1000.0, "R"=100.0, "G"=100.0, "B"=100.0}, {"X"=3300.0, "Y"=3830.0, "Object type"=2.0, "Radius"=0.0, "Width"=200.0, "Height"=20.0, "Theta"=0.0, "HP"=-1000.0, "R"=100.0, "G"=100.0, "B"=100.0}, {"X"=3500.0, "Y"=3830.0, "Object type"=2.0, "Radius"=0.0, "Width"=200.0, "Height"=20.0, "Theta"=0.0, "HP"=-1000.0, "R"=100.0, "G"=100.0, "B"=100.0}, {"X"=3700.0, "Y"=3830.0, "Object type"=2.0, "Radius"=0.0, "Width"=200.0, "Height"=20.0, "Theta"=0.0, "HP"=-1000.0, "R"=100.0, "G"=100.0, "B"=100.0}, {"X"=3900.0, "Y"=3830.0, "Object type"=2.0, "Radius"=0.0, "Width"=200.0, "Height"=20.0, "Theta"=0.0, "HP"=-1000.0, "R"=100.0, "G"=100.0, "B"=100.0}, {"X"=10.0, "Y"=120.0, "Object type"=2.0, "Radius"=0.0, "Width"=200.0, "Height"=20.0, "Theta"=1.57, "HP"=-1000.0, "R"=100.0, "G"=100.0, "B"=100.0}, {"X"=10.0, "Y"=320.0, "Object type"=2.0, "Radius"=0.0, "Width"=200.0, "Height"=20.0, "Theta"=1.57, "HP"=-1000.0, "R"=100.0, "G"=100.0, "B"=100.0}, {"X"=10.0, "Y"=520.0, "Object type"=2.0, "Radius"=0.0, "Width"=200.0, "Height"=20.0, "Theta"=1.57, "HP"=-1000.0, "R"=100.0, "G"=100.0, "B"=100.0}, {"X"=10.0, "Y"=720.0, "Object type"=2.0, "Radius"=0.0, "Width"=200.0, "Height"=20.0, "Theta"=1.57, "HP"=-1000.0, "R"=100.0, "G"=100.0, "B"=100.0}, {"X"=10.0, "Y"=920.0, "Object type"=2.0, "Radius"=0.0, "Width"=200.0, "Height"=20.0, "Theta"=1.57, "HP"=-1000.0, "R"=100.0, "G"=100.0, "B"=100.0}, {"X"=10.0, "Y"=1120.0, "Object type"=2.0, "Radius"=0.0, "Width"=200.0, "Height"=20.0, "Theta"=1.57, "HP"=-1000.0, "R"=100.0, "G"=100.0, "B"=100.0}, {"X"=10.0, "Y"=1320.0, "Object type"=2.0, "Radius"=0.0, "Width"=200.0, "Height"=20.0, "Theta"=1.57, "HP"=-1000.0, "R"=100.0, "G"=100.0, "B"=100.0}, {"X"=10.0, "Y"=1520.0, "Object type"=2.0, "Radius"=0.0, "Width"=200.0, "Height"=20.0, "Theta"=1.57, "HP"=-1000.0, "R"=100.0, "G"=100.0, "B"=100.0}, {"X"=10.0, "Y"=1720.0, "Object type"=2.0, "Radius"=0.0, "Width"=200.0, "Height"=20.0, "Theta"=1.57, "HP"=-1000.0, "R"=100.0, "G"=100.0, "B"=100.0}, {"X"=10.0, "Y"=1920.0, "Object type"=2.0, "Radius"=0.0, "Width"=200.0, "Height"=20.0, "Theta"=1.57, "HP"=-1000.0, "R"=100.0, "G"=100.0, "B"=100.0}, {"X"=10.0, "Y"=2120.0, "Object type"=2.0, "Radius"=0.0, "Width"=200.0, "Height"=20.0, "Theta"=1.57, "HP"=-1000.0, "R"=100.0, "G"=100.0, "B"=100.0}, {"X"=10.0, "Y"=2320.0, "Object type"=2.0, "Radius"=0.0, "Width"=200.0, "Height"=20.0, "Theta"=1.57, "HP"=-1000.0, "R"=100.0, "G"=100.0, "B"=100.0}, {"X"=10.0, "Y"=2520.0, "Object type"=2.0, "Radius"=0.0, "Width"=200.0, "Height"=20.0, "Theta"=1.57, "HP"=-1000.0, "R"=100.0, "G"=100.0, "B"=100.0}, {"X"=10.0, "Y"=2720.0, "Object type"=2.0, "Radius"=0.0, "Width"=200.0, "Height"=20.0, "Theta"=1.57, "HP"=-1000.0, "R"=100.0, "G"=100.0, "B"=100.0}, {"X"=10.0, "Y"=2920.0, "Object type"=2.0, "Radius"=0.0, "Width"=200.0, "Height"=20.0, "Theta"=1.57, "HP"=-1000.0, "R"=100.0, "G"=100.0, "B"=100.0}, {"X"=10.0, "Y"=3120.0, "Object type"=2.0, "Radius"=0.0, "Width"=200.0, "Height"=20.0, "Theta"=1.57, "HP"=-1000.0, "R"=100.0, "G"=100.0, "B"=100.0}, {"X"=10.0, "Y"=3320.0, "Object type"=2.0, "Radius"=0.0, "Width"=200.0, "Height"=20.0, "Theta"=1.57, "HP"=-1000.0, "R"=100.0, "G"=100.0, "B"=100.0}, {"X"=10.0, "Y"=3520.0, "Object type"=2.0, "Radius"=0.0, "Width"=200.0, "Height"=20.0, "Theta"=1.57, "HP"=-1000.0, "R"=100.0, "G"=100.0, "B"=100.0}, {"X"=10.0, "Y"=3720.0, "Object type"=2.0, "Radius"=0.0, "Width"=200.0, "Height"=20.0, "Theta"=1.57, "HP"=-1000.0, "R"=100.0, "G"=100.0, "B"=100.0}, {"X"=3830.0, "Y"=120.0, "Object type"=2.0, "Radius"=0.0, "Width"=200.0, "Height"=20.0, "Theta"=1.57, "HP"=-1000.0, "R"=100.0, "G"=100.0, "B"=100.0}, {"X"=3830.0, "Y"=320.0, "Object type"=2.0, "Radius"=0.0, "Width"=200.0, "Height"=20.0, "Theta"=1.57, "HP"=-1000.0, "R"=100.0, "G"=100.0, "B"=100.0}, {"X"=3830.0, "Y"=520.0, "Object type"=2.0, "Radius"=0.0, "Width"=200.0, "Height"=20.0, "Theta"=1.57, "HP"=-1000.0, "R"=100.0, "G"=100.0, "B"=100.0}, {"X"=3830.0, "Y"=720.0, "Object type"=2.0, "Radius"=0.0, "Width"=200.0, "Height"=20.0, "Theta"=1.57, "HP"=-1000.0, "R"=100.0, "G"=100.0, "B"=100.0}, {"X"=3830.0, "Y"=920.0, "Object type"=2.0, "Radius"=0.0, "Width"=200.0, "Height"=20.0, "Theta"=1.57, "HP"=-1000.0, "R"=100.0, "G"=100.0, "B"=100.0}, {"X"=3830.0, "Y"=1120.0, "Object type"=2.0, "Radius"=0.0, "Width"=200.0, "Height"=20.0, "Theta"=1.57, "HP"=-1000.0, "R"=100.0, "G"=100.0, "B"=100.0}, {"X"=3830.0, "Y"=1320.0, "Object type"=2.0, "Radius"=0.0, "Width"=200.0, "Height"=20.0, "Theta"=1.57, "HP"=-1000.0, "R"=100.0, "G"=100.0, "B"=100.0}, {"X"=3830.0, "Y"=1520.0, "Object type"=2.0, "Radius"=0.0, "Width"=200.0, "Height"=20.0, "Theta"=1.57, "HP"=-1000.0, "R"=100.0, "G"=100.0, "B"=100.0}, {"X"=3830.0, "Y"=1720.0, "Object type"=2.0, "Radius"=0.0, "Width"=200.0, "Height"=20.0, "Theta"=1.57, "HP"=-1000.0, "R"=100.0, "G"=100.0, "B"=100.0}, {"X"=3830.0, "Y"=1920.0, "Object type"=2.0, "Radius"=0.0, "Width"=200.0, "Height"=20.0, "Theta"=1.57, "HP"=-1000.0, "R"=100.0, "G"=100.0, "B"=100.0}, {"X"=3830.0, "Y"=2120.0, "Object type"=2.0, "Radius"=0.0, "Width"=200.0, "Height"=20.0, "Theta"=1.57, "HP"=-1000.0, "R"=100.0, "G"=100.0, "B"=100.0}, {"X"=3830.0, "Y"=2320.0, "Object type"=2.0, "Radius"=0.0, "Width"=200.0, "Height"=20.0, "Theta"=1.57, "HP"=-1000.0, "R"=100.0, "G"=100.0, "B"=100.0}, {"X"=3830.0, "Y"=2520.0, "Object type"=2.0, "Radius"=0.0, "Width"=200.0, "Height"=20.0, "Theta"=1.57, "HP"=-1000.0, "R"=100.0, "G"=100.0, "B"=100.0}, {"X"=3830.0, "Y"=2720.0, "Object type"=2.0, "Radius"=0.0, "Width"=200.0, "Height"=20.0, "Theta"=1.57, "HP"=-1000.0, "R"=100.0, "G"=100.0, "B"=100.0}, {"X"=3830.0, "Y"=2920.0, "Object type"=2.0, "Radius"=0.0, "Width"=200.0, "Height"=20.0, "Theta"=1.57, "HP"=-1000.0, "R"=100.0, "G"=100.0, "B"=100.0}, {"X"=3830.0, "Y"=3120.0, "Object type"=2.0, "Radius"=0.0, "Width"=200.0, "Height"=20.0, "Theta"=1.57, "HP"=-1000.0, "R"=100.0, "G"=100.0, "B"=100.0}, {"X"=3830.0, "Y"=3320.0, "Object type"=2.0, "Radius"=0.0, "Width"=200.0, "Height"=20.0, "Theta"=1.57, "HP"=-1000.0, "R"=100.0, "G"=100.0, "B"=100.0}, {"X"=3830.0, "Y"=3520.0, "Object type"=2.0, "Radius"=0.0, "Width"=200.0, "Height"=20.0, "Theta"=1.57, "HP"=-1000.0, "R"=100.0, "G"=100.0, "B"=100.0}, {"X"=3830.0, "Y"=3720.0, "Object type"=2.0, "Radius"=0.0, "Width"=200.0, "Height"=20.0, "Theta"=1.57, "HP"=-1000.0, "R"=100.0, "G"=100.0, "B"=100.0}], "Max Player ID number"=20, "Moving Object"=T1 {"X"=3690.0, "Y"=450.0, "Object type"=0.0, "Move info"=0.0, "Vector scalar"=0.0, "Vector theta"=0.0}) -> ()  [unwired: 2 out]
    n6 = Subtract(x=w5, y=w6) -> (x-y=w10:dbl)
    n7 = Divide(x=1.0, y=w10) -> (x/y=→"Hz":dbl)
  }
